vi "__Create New Directory Dialog.vi"(7 "FileManager Data":T1, 8 "error in (no error)":errorcluster) -> (0 "error out":errorcluster)   [LabVIEW 2011]
doc: "This VI launches a pop-up dialog for creating a new directory on the local system."
uses:
  __File manager Data type.ctl
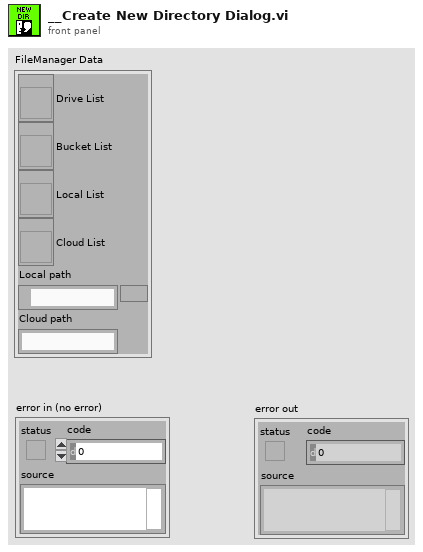
[diagram p1: front panel]
types:
  T1 = typedef "__File manager Data type.ctl" = cluster{"Drive List":refnum<vi>, "Bucket List":refnum<vi>, "Local List":refnum<vi>, "Cloud List":refnum<vi>, "Local path":path, "Cloud path":string}
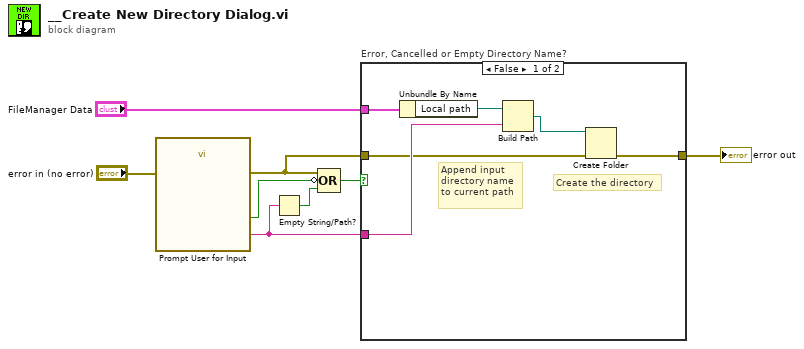
[diagram p0: block diagram]
diagram:
  n1 = call "Prompt User for Input"("error in (no error)"="error in (no error)") -> ("Directory Name"=w4:string, "OK"=w7:bool, "error out"=w2:errorcluster)  [unwired: 16 in]
  n2 = Empty String/Path?(string/path=w4) -> (empty?=w3:bool)
  n3 = Compound Arithmetic op=OR(w2, invert w7, w3) -> (w6:bool)
  n4 = case "Error, Cancelled or Empty Directory Name?" shown="False" w6 {
    tunnel: w4 -> [w12 _]
    tunnel: "FileManager Data" -> [w14 _]
    tunnel: w2 -> [w10 w15]
    tunnel: [w9 w15] -> w1
    frame False {
      # "Append input\ndirectory name\nto current path"
      # "Create the directory"
      n5 = Unbundle By Name(w14) -> ("Local path"=w13:path)
      n6 = Build Path(base path=w13, name or relative path=w12) -> (appended path=w11:path)
      n7 = Create Folder(path (use dialog)=w11, error in=w10) -> (error out=w9:errorcluster)  [unwired: 1 in, 2 out]
    }
    frame True {
      # "Do nothing"
    }
  }
  "error out" <- w1
